vi "HemisphereFlashingTest.vi"() -> ()   [LabVIEW 2013]
uses:
  <vilib>/Instr/_visa.llb/VISA Configure Serial Port (Instr).vi
panel:
  out "error out":errorcluster
  out "read buffer":string
  in  "Input\nbuffer size":u32=4096
  in  "error in (no error)":errorcluster
  in  "VISA Refnum in":refnum<visa-resource-name>
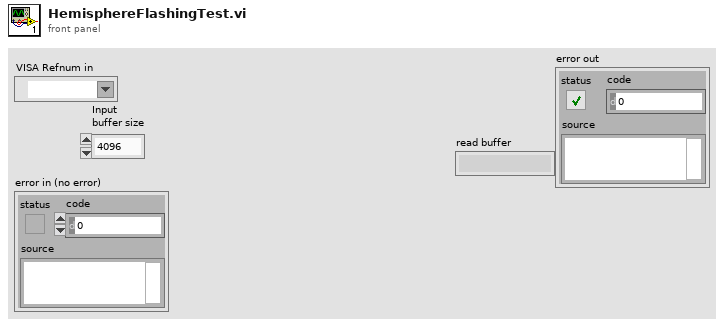
[diagram p1: front panel]
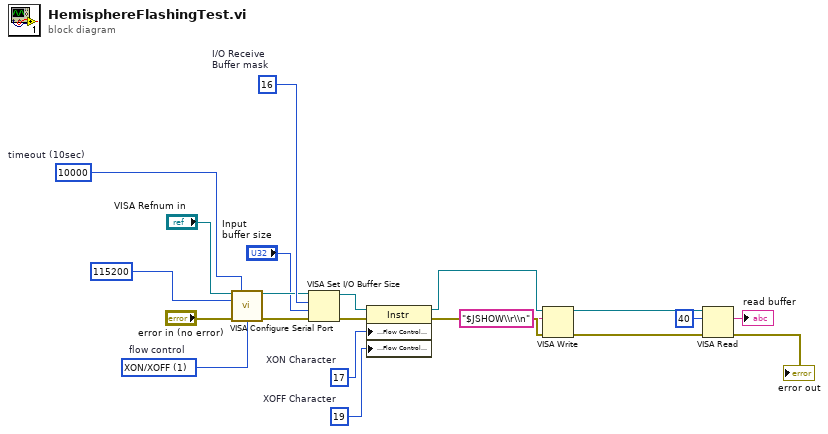
[diagram p0: block diagram]
diagram:
  w18 = u32 10000  # timeout (10sec)
  w15 = u8 19  # XOFF Character
  w14 = u8 17  # XON Character
  w19 = u16 16  # I/O Receive Buffer mask
  w10 = u16 1 items=["None"=0, "XON/XOFF"=1, "RTS/CTS"=2, "DTR/DSR"=4]  # flow control
  n1 = call-poly "VISA Configure Serial Port"("VISA resource name"="VISA Refnum in", "timeout (10sec)"=w18, "baud rate (9600)"=u32 115200, "error in (no error)"="error in (no error)", "flow control (0:none)"=w10) -> ("VISA resource name out"=w16:refnum<visa-resource-name>, "error out"=w17:errorcluster)  [unwired: 9 in]
  n2 = VISA Set I/O Buffer Size(VISA resource name=w16, mask (16)=w19, size (4096)="Input\nbuffer size", error in (no error)=w17) -> (VISA resource name out=w12:refnum<visa-resource-name>, error out=w13:errorcluster)
  n3 = property class="Instr"(reference=w12, error in=w13, "Serial Settings:Flow Control XON Character"=w14, "Serial Settings:Flow Control XOFF Character"=w15) -> (reference out=w8:refnum<visa-resource-name>, error out=w7:errorcluster)
  n4 = VISA Write(VISA resource name=w8, write buffer="$JSHOW\\r\\n", error in (no error)=w7) -> (VISA resource name out=w5:refnum<visa-resource-name>, error out=w3:errorcluster)  [unwired: 1 out]
  n5 = VISA Read(VISA resource name=w5, byte count=u32 40, error in (no error)=w3) -> (read buffer=→"read buffer":string, error out=→"error out":errorcluster)  [unwired: 2 out]
